vi "AdjustPuffTimings.vi"(11 "Input Trigger Data":T3) -> (3 "Output Trigger Data":T3)   [LabVIEW 2016]
uses:
  Ctrl_Signal.ctl
  Ctrl_Signal_Map.ctl
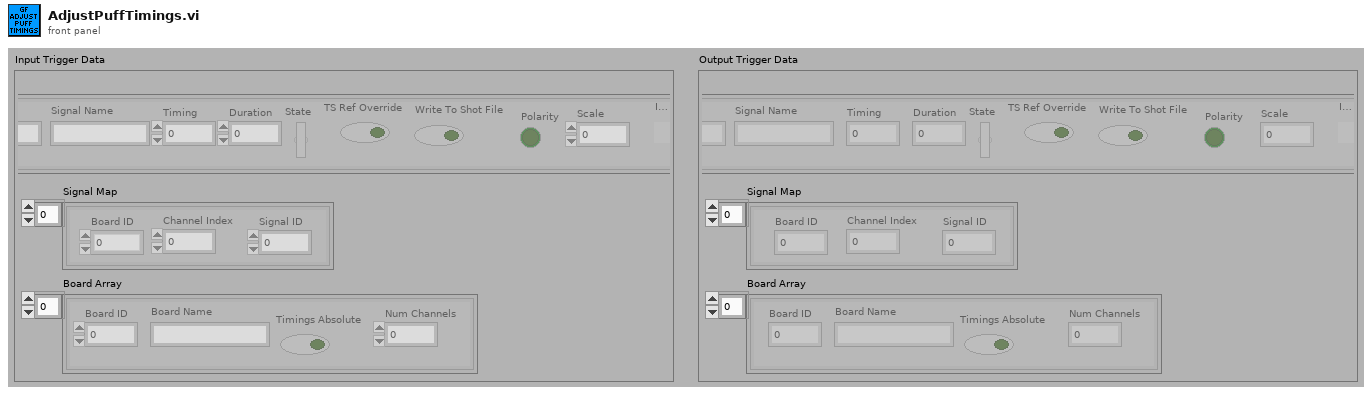
[diagram p1: front panel]
types:
  T1 = typedef "Ctrl_Signal.ctl" = cluster{"Signal Name":string, "Timing":dbl, "Duration":dbl, "State":bool, "TS Ref Override":bool, "Write To Shot File":bool, "Polarity":bool, "Signal ID":dbl, "Scale":dbl, "IsDelay":bool}
  T2 = typedef "Ctrl_Signal_Map.ctl" = cluster{"Channel Index":dbl, "Board ID":dbl, "Signal ID":dbl}
  T3 = cluster{"Signal Array":T1[], "Signal Map":T2[], "Board Array":cluster{"Board ID":dbl, "Board Name":string, "Timings Absolute":bool, "Num Channels":dbl}[]}
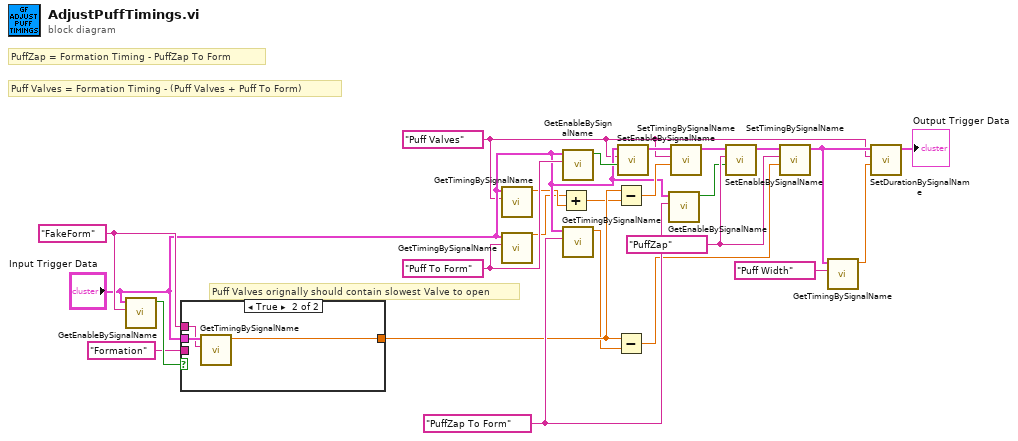
[diagram p0: block diagram]
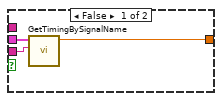
[diagram p2: hidden frame]
diagram:
  w14 = "PuffZap" ("Signal Name")
  w1 = "Puff Valves" ("Signal Name")
  w21 = "PuffZap To Form" ("Signal Name")
  w20 = "Puff To Form" ("Signal Name")
  w23 = "FakeForm" ("Signal Name")
  # "Puff Valves orignally should contain slowest Valve to open"
  # "PuffZap = Formation Timing - PuffZap To Form"
  # "Puff Valves = Formation Timing - (Puff Valves + Puff To Form)"
  n1 = call "GetEnableBySignalName.vi"("Signal Name"=w23, "Trigger Data"="Input Trigger Data") -> ("Signal Enabled"=w24:bool)  [unwired: 9 in]
  n2 = case shown="True" w24 {
    tunnel: "Input Trigger Data" -> [w27 w30]
    tunnel: w23 -> [_ w29]
    tunnel: "Formation" ("Signal Name") -> [w26 _]
    tunnel: [w25 w28] -> w12
    frame False {
      n3 = call "GetTimingBySignalName.vi"("Signal Name"=w26, "Trigger Data"=w27) -> ("Timing"=w25:dbl)  [unwired: 9 in]
    }
    frame True {
      n4 = call "GetTimingBySignalName.vi"("Signal Name"=w29, "Trigger Data"=w30) -> ("Timing"=w28:dbl)  [unwired: 9 in]
    }
  }
  n5 = call "GetTimingBySignalName.vi"("Signal Name"=w1, "Trigger Data"="Input Trigger Data") -> ("Timing"=w8:dbl)  [unwired: 9 in]
  n6 = call "GetTimingBySignalName.vi"("Signal Name"=w20, "Trigger Data"="Input Trigger Data") -> ("Timing"=w7:dbl)  [unwired: 9 in]
  n7 = Add(x=w7, y=w8) -> (x+y=w6:dbl)
  n8 = call "GetEnableBySignalName.vi"("Signal Name"=w20, "Trigger Data"="Input Trigger Data") -> ("Signal Enabled"=w16:bool)  [unwired: 9 in]
  n9 = call "GetTimingBySignalName.vi"("Signal Name"=w21, "Trigger Data"="Input Trigger Data") -> ("Timing"=w11:dbl)  [unwired: 9 in]
  n10 = Subtract(x=w12, y=w6) -> (x-y=w15:dbl)
  n11 = Subtract(x=w12, y=w11) -> (x-y=w10:dbl)
  n12 = call "SetEnableBySignalName.vi"("State"=w16, "Signal Name"=w1, "Trigger Data Input"="Input Trigger Data") -> ("Trigger Data Output"=w19:T3)  [unwired: 8 in]
  n13 = call "GetEnableBySignalName.vi"("Signal Name"=w21, "Trigger Data"="Input Trigger Data") -> ("Signal Enabled"=w13:bool)  [unwired: 9 in]
  n14 = call "SetTimingBySignalName.vi"("Timing"=w15, "Signal Name"=w1, "Trigger Data Input"=w19) -> ("Trigger Data Output"=w18:T3)  [unwired: 8 in]
  n15 = call "SetEnableBySignalName.vi"("State"=w13, "Signal Name"=w14, "Trigger Data Input"=w18) -> ("Trigger Data Output"=w17:T3)  [unwired: 8 in]
  n16 = call "SetTimingBySignalName.vi"("Timing"=w10, "Signal Name"=w14, "Trigger Data Input"=w17) -> ("Trigger Data Output"=w4:T3)  [unwired: 8 in]
  n17 = call "GetTimingBySignalName.vi"("Signal Name"="Puff Width", "Trigger Data"=w4) -> ("Timing"=w2:dbl)  [unwired: 9 in]
  n18 = call "SetDurationBySignalName.vi"("Duration"=w2, "Signal Name"=w1, "Trigger Data Input"=w4) -> ("Trigger Data Output"=→"Output Trigger Data":T3)  [unwired: 8 in]
